vi "volumetric_efficiency_calculate.vi"(6 "P amb":dbl, 9 "ECU RPM":dbl, 10 "T HFM":dbl, 11 "Bovito":dbl[](array[numeric])) -> (3 "ve":dbl)   [LabVIEW 2014]
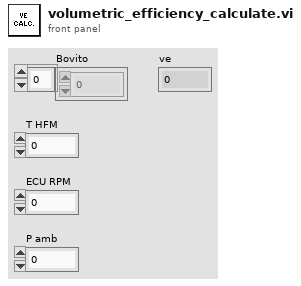
[diagram p1: front panel]
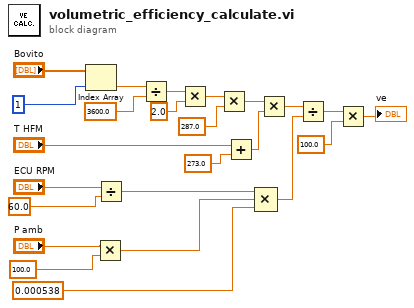
[diagram p0: block diagram]
diagram:
  n1 = Index Array(array="Bovito", index=1) -> (element=w3:dbl)
  n2 = Multiply(x="P amb", y=100.0) -> (x*y=w23:dbl)
  n3 = Divide(x="ECU RPM", y=60.0) -> (x/y=w20:dbl)
  n4 = Divide(x=w3, y=3600.0) -> (x/y=w5:dbl)
  n5 = Multiply(x=w5, y=2.0) -> (x*y=w7:dbl)
  n6 = Multiply(x=w7, y=287.0) -> (x*y=w9:dbl)
  n7 = Add(x="T HFM", y=273.0) -> (x+y=w12:dbl)
  n8 = Compound Arithmetic op=MULTIPLY(w20, w23, 0.000538) -> (w14:dbl)
  n9 = Multiply(x=w9, y=w12) -> (x*y=w13:dbl)
  n10 = Divide(x=w13, y=w14) -> (x/y=w15:dbl)
  n11 = Multiply(x=w15, y=100.0) -> (x*y=→"ve":dbl)
